vi "LVClass_HasoEngine do new lens.vi"(0 "HasoEngine in":refnum<class "HasoEngine.lvclass">, 11 "error in (no error)":errorcluster) -> (4 "HasoEngine out":refnum<class "HasoEngine.lvclass">, 15 "error out":errorcluster)   [LabVIEW 2020, in "HasoEngine.lvclass"]
doc: "Reset spots detection. In particular, reinitialize the spots tracking.\n\n--------------------------------------------------------------------------------\n\n<B>HasoEngine </B> : HasoEngine object.\n<B>ErrorIn </B> : Error\n<B>ErrorOut </B> : Error\n\n--------------------------------------------------------------------------------"
uses:
  HasoEngine.lvclass
  HasoEngine.lvclass/HasoEngine.ctl
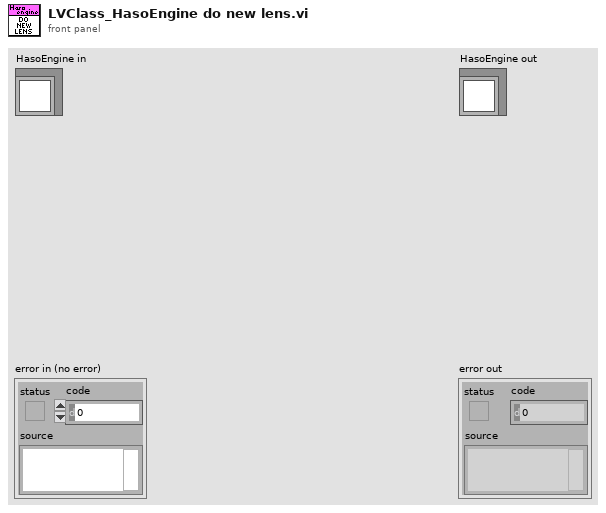
[diagram p1: front panel]
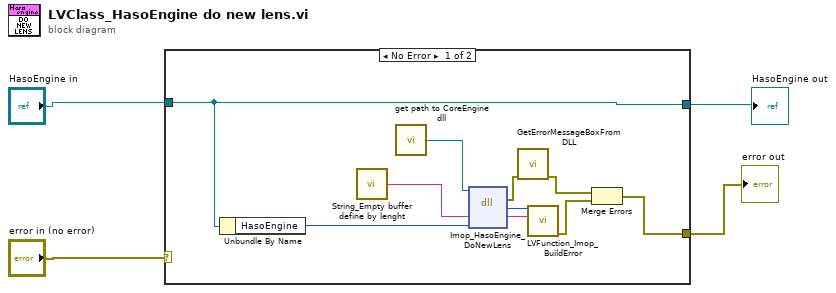
[diagram p0: block diagram]
diagram:
  n1 = case shown="No Error" "error in (no error)" {
    selector: "error in (no error)" -> [_ w15]
    tunnel: "HasoEngine in" -> [w9 w16]
    tunnel: [w9 w16] -> w1
    tunnel: [w5 w15] -> w2
    frame No Error {
      n2 = Unbundle By Name(w9) -> ("HasoEngine"=w8:i32)
      n3 = call "String_Empty buffer define by lenght.vi"() -> ("Empty buffer"=w14:string)  [unwired: 1 in]
      n4 = call "get path to CoreEngine dll.vi"() -> ("path to c_interface_vc100.dll"=w11:path)  [unwired: 12 in, 3 out]
      n5 = dll-call lib="D:/2_trunk/Soft_haso/ImOpCoreEngine4_LV2011/DLLs/ImopEngine4_vc100.dll" fn="Imop_HasoEngine_DoNewLens"(path in=w11, "message"=w14, "objet"=w8) -> (error out=w10:errorcluster, "return type"=w12:i32, "message"=w13:string)  [unwired: 3 in, 1 out]
      n6 = call "GetErrorMessageBoxFromDLL.vi"("error IN"=w10) -> ("error OUT"=w7:errorcluster)  [unwired: 10 in]
      n7 = call "LVFunction_Imop_BuildError.vi"("code"=w12, "String to Prepend to source (\"\")"=w13) -> ("error out"=w6:errorcluster)  [unwired: 13 in]
      n8 = Merge Errors(w7, w6) -> (w5:errorcluster)
    }
    frame Error {
    }
  }
  "error out" <- w2
  "HasoEngine out" <- w1
